vi "ActorCoreEvent.vi"(8 "error in (no error)":errorcluster, 10 "ActorCoreMessage":string, 11 "EventRecorder in":refnum<class "EventRecorder.lvclass">) -> (0 "error out":errorcluster, 3 "EventRecorder out":refnum<class "EventRecorder.lvclass">)   [LabVIEW 2019, in "EventRecorder.lvlib" / "EventRecorder.lvclass"]
uses:
  EventRecorder.lvclass
  EventRecorder.lvclass/EventRecorder.ctl
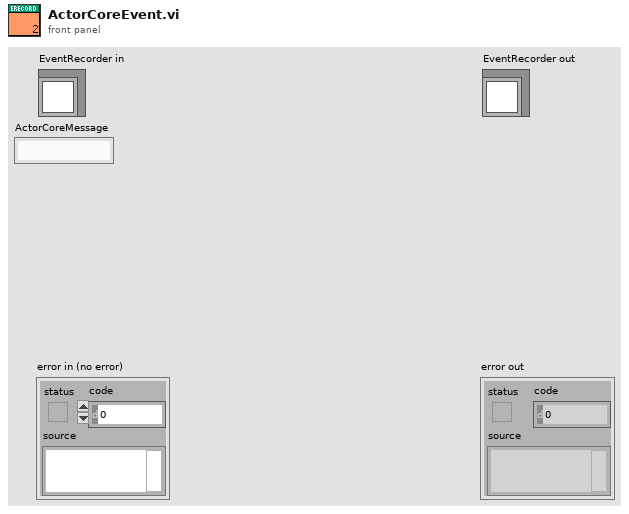
[diagram p1: front panel]
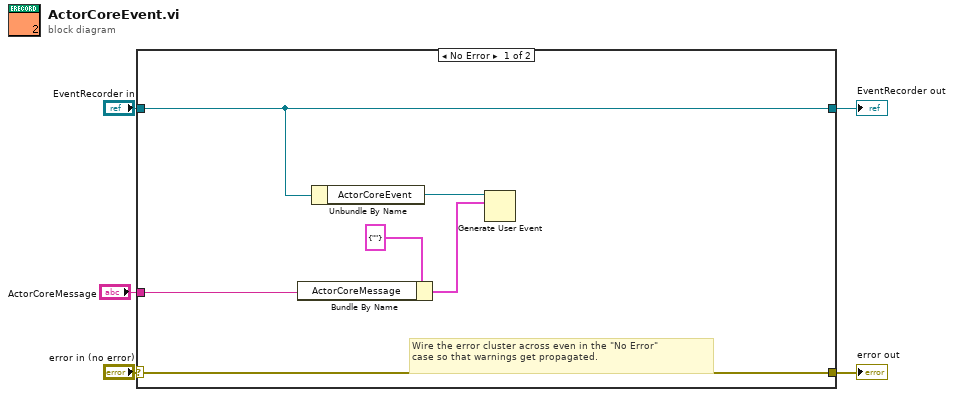
[diagram p0: block diagram]
diagram:
  n1 = case shown="No Error" "error in (no error)" {
    selector: "error in (no error)" -> [w11 w13]
    tunnel: [w11 w13] -> w4
    tunnel: [w10 w12] -> w2
    tunnel: "EventRecorder in" -> [w10 w12]
    tunnel: "ActorCoreMessage" -> [w6 _]
    frame No Error {
      # "Wire the error cluster across even in the \"No Error\"\ncase so that warnings get propagated."
      n2 = Bundle By Name(cluster=cluster{"ActorCoreMessage":string} {"ActorCoreMessage"=""} ("event data"), "ActorCoreMessage"=w6) -> (w7:cluster{"ActorCoreMessage":string})
      n3 = Unbundle By Name(w10) -> ("ActorCoreEvent"=w9:refnum<user-event>)
      n4 = Generate User Event(user event=w9, event data cluster=w7) -> ()  [unwired: 2 in, 2 out]
    }
    frame Error {
    }
  }
  "error out" <- w4
  "EventRecorder out" <- w2
